vi "Launcher.vi"() -> ()   [LabVIEW 2022 SP3]
uses:
  <vilib>/ErrorRing/Error Ring.xnode
panel:
  out "error out":errorcluster
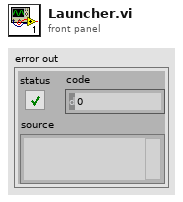
[diagram p1: front panel]
types:
  T1 = cluster{"Minimum Splash Screen Time (ms)":u32, "Splash Screen Start Time (ms)":u32}
  T2 = enum32{"Invalid", "Standard", "Closed", "Hidden", "Minimized", "Maximized"}
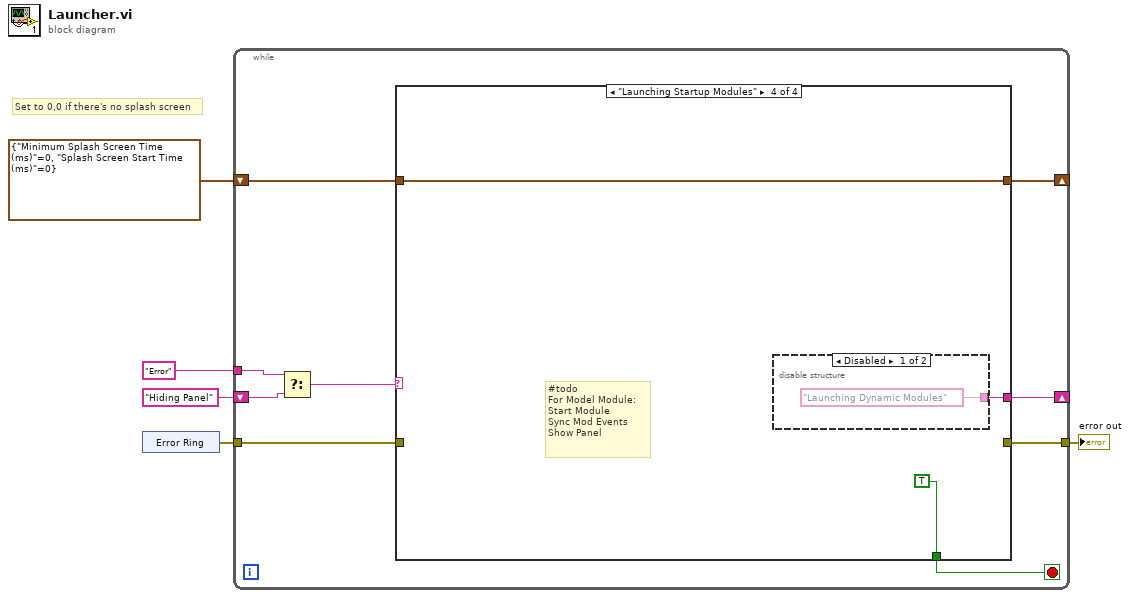
[diagram p0: block diagram]
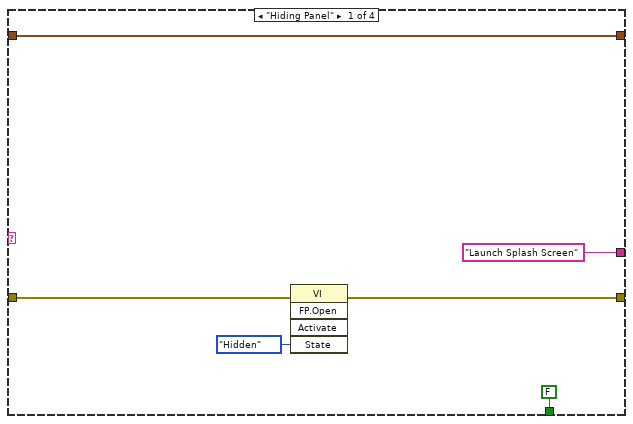
[diagram p2: hidden frame]
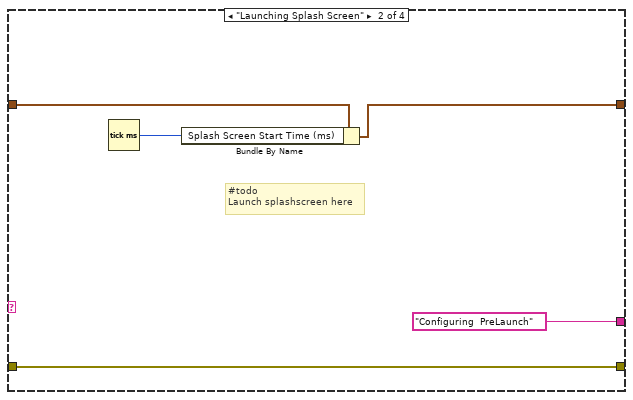
[diagram p3: hidden frame]
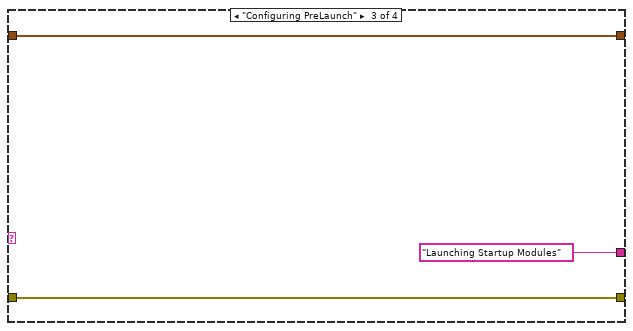
[diagram p4: hidden frame]
diagram:
  # "Set to 0,0 if there's no splash screen"
  n1 = xnode "Error Ring"() -> ("error out"=w3:errorcluster)
  n2 = while {
    tunnel: "Error" -> [w14]
    tunnel: w3 -> [w11]
    tunnel: [w10] -> w2
    shift-right: [w9] -> _
    shift-left: "Hiding Panel" -> [w13]
    shift-right: [w7] -> _
    shift-left: T1 {"Minimum Splash Screen Time (ms)"=0, "Splash Screen Start Time (ms)"=0} -> [w8]
    stop <- w6 stop-if-true
    n3 = Select(t=w14, f=w13) -> (s? t:f=w12:string)  [unwired: 1 in]
    n4 = case shown="\"Launching Startup Modules\"" w12 {
      tunnel: w11 -> [w19 w25 w27 _]
      tunnel: [w18 w25 w27 _] -> w10
      tunnel: ["Launch Splash Screen" "Configuring  PreLaunch" "Launching Startup Modules" w31] -> w9
      tunnel: w8 -> [w16 w23 w28 w30]
      tunnel: [w16 w21 w28 w30] -> w7
      tunnel: [FALSE _ _ TRUE] -> w6
      frame "Hiding Panel" {
        n5 = invoke class="VI" method="FP.Open"(error in=w19, "State"=T2."Hidden") -> (error out=w18:errorcluster)  [unwired: 3 in, 4 out]
      }
      frame "Launching Splash Screen" {
        # "#todo\nLaunch splashscreen here"
        n6 = Tick Count (ms)() -> (millisecond timer value=w22:u32)
        n7 = Bundle By Name(cluster=w23, "Splash Screen Start Time (ms)"=w22) -> (w21:T1)
      }
      frame "Configuring PreLaunch" {
      }
      frame "Launching Startup Modules" {
        # "#todo\nFor Model Module:\nStart Module\nSync Mod Events\nShow Panel"
        n8 = disable-structure shown="Disabled" {
          disable-tunnel: ["Launching Dynamic Modules" _] -> w31
          frame Disabled {
          }
          frame Enabled {
          }
        }
      }
    }
  }
  "error out" <- w2
